vi "as56007.vi"() -> ()   [LabVIEW 2025]
uses:
  <vilib>/Instr/_visa.llb/VISA Configure Serial Port (Instr).vi
  <vilib>/ptbypt/NI_PtbyPt.lvlib
panel:
  out "Aceleração (cm/s²)":dbl
  out "Velocidade (cm/s)":dbl
  in  "Gravar":bool
  out "Aceleração da Abertura":dbl(graph)
  out "Velocidade de Abertura":dbl(graph)
  out "Gráfico de Abertura":dbl(graph)
  out "Abertura Linear (cm)":dbl
  in  "Raio da Mandíbula (cm)":dbl=6.0 min=6.0 max=14.0 step=0.1
  out "Cabeça do Paciente":picture
  in  "stop":bool
  in  "VISA resource name":refnum<visa-resource-name>
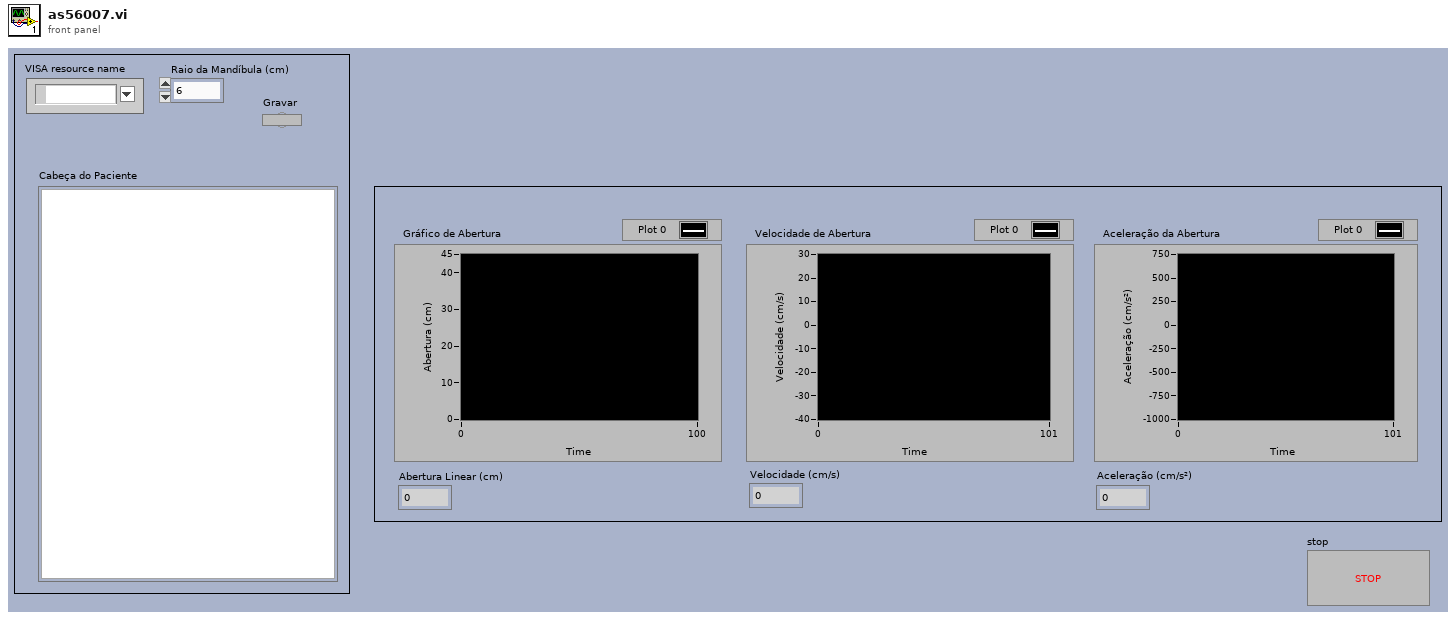
[diagram p1: front panel]
types:
  T1 = enum16{"open", "replace", "create", "open or create", "replace or create", "replace or create with confirmation"}
  T2 = typedef "imagedata.ctl" = cluster{"image type":i32, "image depth":i32, "image":u8[], "mask":u8[], "colors":u32[], "Rectangle":cluster{"left":i16, "top":i16, "right":i16, "bottom":i16}}
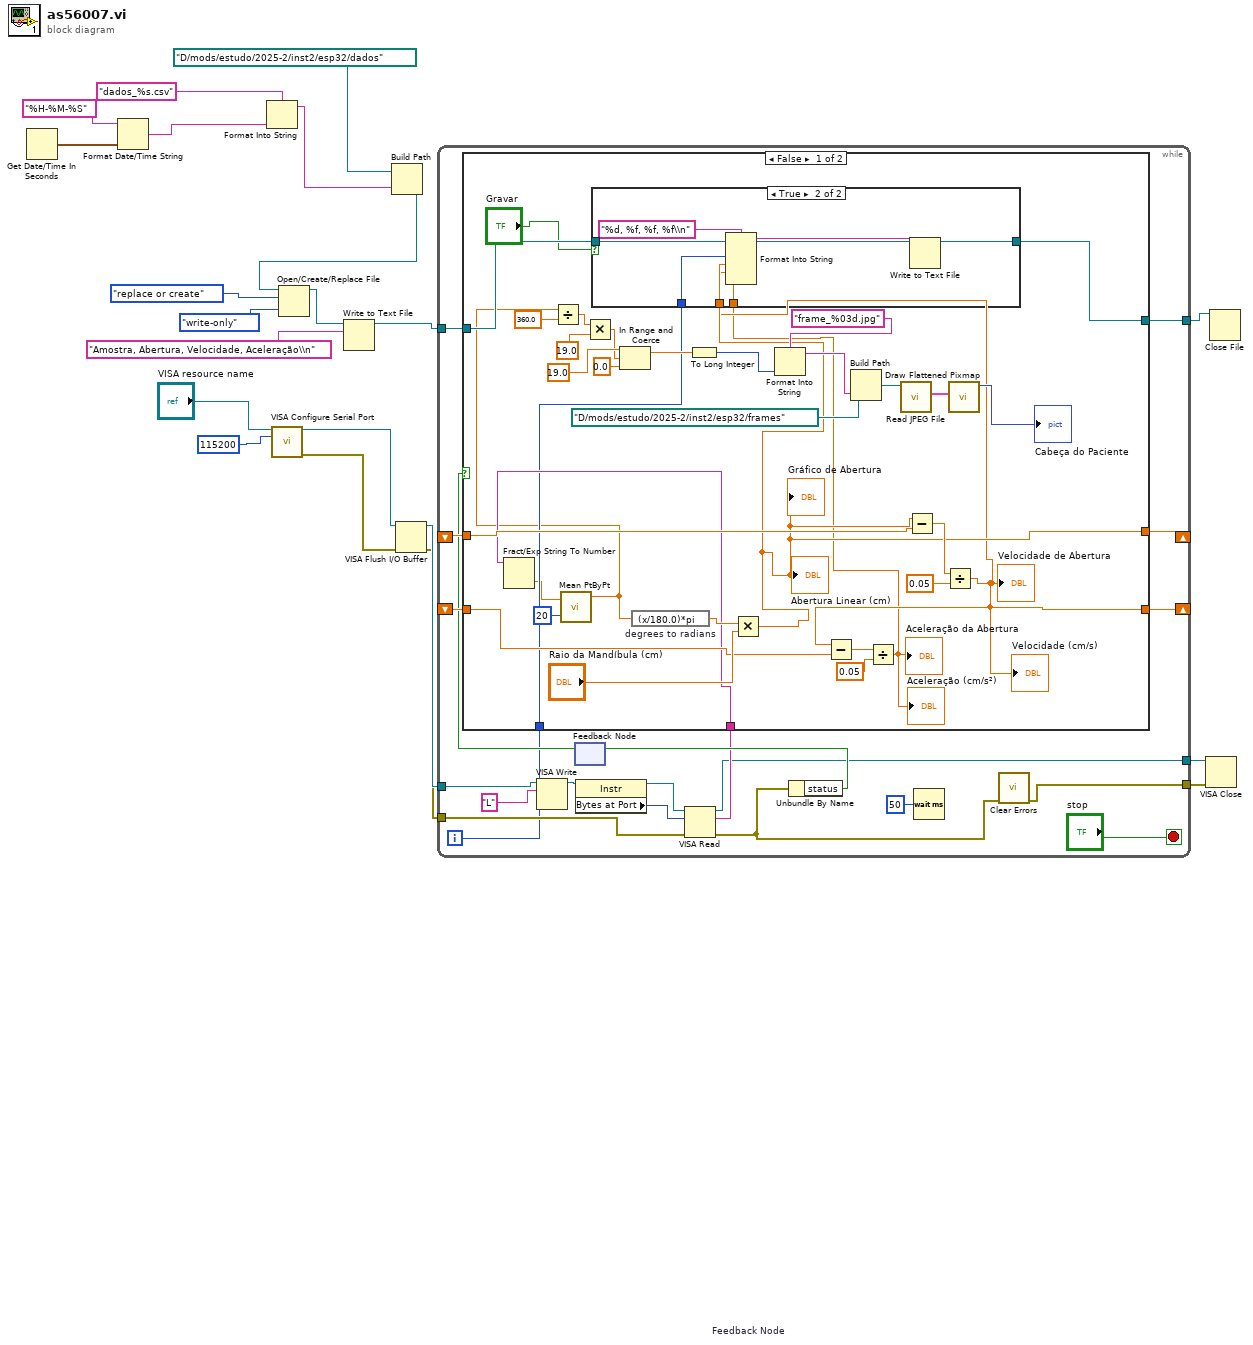
[diagram p0: block diagram]
diagram:
  n1 = Get Date/Time In Seconds() -> (seconds since 1Jan1904=w7:timestamp)
  n2 = Format Date/Time String(time format string (%c)="%H-%M-%S", seconds (now)=w7) -> (date/time string=w5:string)  [unwired: 1 in]
  n3 = Format Into String "Format Into String"(format string="dados_%s.csv", w5) -> (resulting string=w1:string)  [unwired: 2 in, 1 out]
  n4 = call-poly "VISA Configure Serial Port"("VISA resource name"="VISA resource name", "baud rate (9600)"=u32 115200) -> ("VISA resource name out"=w21:refnum<visa-resource-name>, "error out"=w20:errorcluster)  [unwired: 12 in]
  n5 = Build Path(base path=path "D:/mods/estudo/2025-2/inst2/esp32/dados", name or relative path=w1) -> (appended path=w3:path)
  n6 = Open/Create/Replace File(file path (use dialog)=w3, operation (0:open)=T1."replace or create", access (0:read/write)=enum16{"read/write", "read-only", "write-only"}."write-only") -> (refnum out=w10:refnum<file>)  [unwired: 3 in, 2 out]
  n7 = Write to Text File(file (use dialog)=w10, text="Amostra, Abertura, Velocidade, Aceleração\\n") -> (refnum out=w9:refnum<file>)  [unwired: 2 in, 2 out]
  n8 = VISA Flush I/O Buffer(VISA resource name=w21, error in (no error)=w20) -> (VISA resource name out=w19:refnum<visa-resource-name>, error out=w18:errorcluster)  [unwired: 1 in]
  n9 = while {
    tunnel: w19 -> [w41]
    tunnel: w18 -> [w40]
    shift-right: [w38] -> _
    shift-left: _ -> [w39]
    shift-right: [w36] -> _
    shift-left: _ -> [w37]
    tunnel: [w30] -> w15
    tunnel: [w29] -> w14
    tunnel: w9 -> [w28]
    tunnel: [w27] -> w11
    i -> [w26]
    stop <- "stop" stop-if-true
    n10 = VISA Write(VISA resource name=w41, write buffer="L") -> (VISA resource name out=w24:refnum<visa-resource-name>)  [unwired: 1 in, 2 out]
    n11 = feedback #1 "Feedback Node"() -> (w34:bool)  [unwired: 1 in]
    n12 = property class="Instr"(reference=w24) -> (reference out=w23:refnum<visa-resource-name>, "Bytes at Port"=w22:u32)  [unwired: 1 in, 1 out]
    n13 = VISA Read(VISA resource name=w23, byte count=w22, error in (no error)=w40) -> (VISA resource name out=w29:refnum<visa-resource-name>, read buffer=w32:string, error out=w33:errorcluster)  [unwired: 1 out]
    n14 = case shown="False" w34 {
      tunnel: w39 -> [w59 w87]
      tunnel: [w45 w87] -> w38
      tunnel: w37 -> [w56 w86]
      tunnel: [w44 w86] -> w36
      tunnel: w32 -> [w53 _]
      tunnel: w28 -> [w51 w85]
      tunnel: [w50 w85] -> w27
      tunnel: w26 -> [w52 _]
      frame False {
        n15 = Fract/Exp String To Number(string=w53) -> (number=w49:dbl)  [unwired: 3 in, 1 out]
        n16 = call <vilib>:"Mean PtByPt.vi"("x"=w49, "sample length"=20) -> ("mean"=w48:dbl)  [unwired: 2 in, 1 out]
        n17 = Divide(x=w48, y=360.0) -> (x/y=w74:dbl)
        n18 = Multiply(x=w74, y=19.0) -> (x*y=w64:dbl)
        n19 = In Range and Coerce(upper limit=19.0, x=w64, lower limit=0.0) -> (coerced(x)=w62:dbl)  [unwired: 1 out]
        n20 = expression code="(x/180.0)*pi" "degrees to radians"(w48) -> (w61:dbl)
        n21 = To Long Integer(number=w62) -> (32bit integer=w66:i32)
        n22 = Multiply(x=w61, y="Raio da Mandíbula (cm)") -> (x*y=w45:dbl)
        "Abertura Linear (cm)" <- w45
        "Gráfico de Abertura" <- w45
        n23 = Format Into String "Format Into String"(format string="frame_%03d.jpg", w66) -> (resulting string=w67:string)  [unwired: 2 in, 1 out]
        n24 = Build Path(base path=path "D:/mods/estudo/2025-2/inst2/esp32/frames", name or relative path=w67) -> (appended path=w71:path)
        n25 = call <vilib>:"Read JPEG File.vi"("path to JPEG file"=w71) -> ("image data"=w70:T2)  [unwired: 8 in, 2 out]
        n26 = Subtract(x=w45, y=w59) -> (x-y=w58:dbl)
        n27 = Divide(x=w58, y=0.05) -> (x/y=w44:dbl)
        "Velocidade de Abertura" <- w44
        "Velocidade (cm/s)" <- w44
        n28 = Subtract(x=w44, y=w56) -> (x-y=w55:dbl)
        n29 = Divide(x=w55, y=0.05) -> (x/y=w43:dbl)
        "Aceleração da Abertura" <- w43
        "Aceleração (cm/s²)" <- w43
        n30 = case shown="True" "Gravar" {
          tunnel: w52 -> [_ w83]
          tunnel: w45 -> [_ w82]
          tunnel: w44 -> [_ w81]
          tunnel: w43 -> [_ w80]
          tunnel: w51 -> [w76 w79]
          tunnel: [w76 w78] -> w50
          frame False {
          }
          frame True {
            n31 = Format Into String "Format Into String"(format string="%d, %f, %f, %f\\n", w83, w82, w81, w80) -> (resulting string=w77:string)  [unwired: 2 in, 1 out]
            n32 = Write to Text File(file (use dialog)=w79, text=w77) -> (refnum out=w78:refnum<file>)  [unwired: 2 in, 2 out]
          }
        }
        n33 = call <vilib>:"Draw Flattened Pixmap.vi"("image data"=w70) -> ("new picture"=→"Cabeça do Paciente":picture)  [unwired: 8 in]
      }
      frame True {
      }
    }
    n34 = Unbundle By Name "Unbundle By Name"(w33) -> ("status"=w35:bool)
    n35 = feedback-in #1(w35) -> ()
    n36 = Wait (ms)(milliseconds to wait=u32 50) -> ()  [unwired: 1 out]
    n37 = call <vilib>:"Clear Errors.vi"("error in (no error)"=w33) -> ("error out"=w30:errorcluster)  [unwired: 5 in, 1 out]
  }
  n38 = VISA Close(VISA resource name=w14, error in (no error)=w15) -> ()  [unwired: 1 out]
  n39 = Close File(refnum=w11) -> ()  [unwired: 1 in, 2 out]
